vi "ReadMessage.vi"(8 "error in (no error)":errorcluster, 11 "StepMotor in":refnum<class "StepMotor.lvclass">) -> (0 "error out":errorcluster, 3 "StepMotor out":refnum<class "StepMotor.lvclass">)   [LabVIEW 2010, in "StepMotor.lvclass"]
doc: "Чтение сообщения из привода СПШ"
uses:
  StepMotor.lvclass
  StepMotor.lvclass/StepMotor.ctl
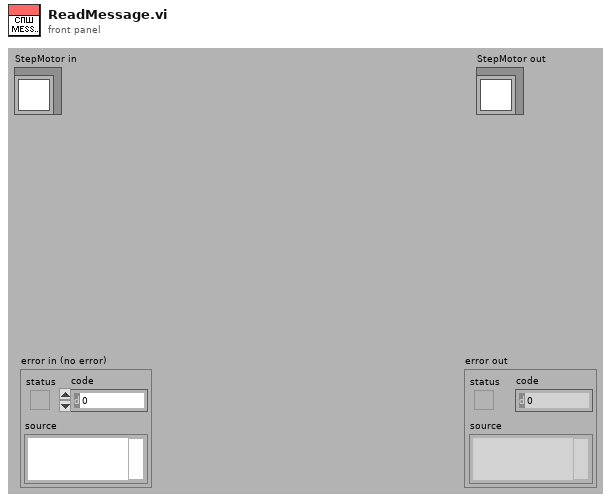
[diagram p1: front panel]
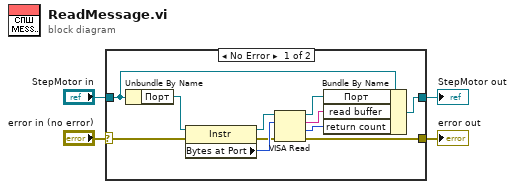
[diagram p0: block diagram]
diagram:
  n1 = case shown="No Error" "error in (no error)" {
    selector: "error in (no error)" -> [w6 w17]
    tunnel: [w8 w17] -> w3
    tunnel: [w14 w16] -> w1
    tunnel: "StepMotor in" -> [w15 w16]
    frame No Error {
      n2 = Unbundle By Name(w15) -> ("Порт"=w5:refnum<visa-resource-name>)
      n3 = property class="Instr"(reference=w5, error in=w6) -> (reference out=w11:refnum<visa-resource-name>, error out=w7:errorcluster, "Bytes at Port"=w10:u32)
      n4 = VISA Read(VISA resource name=w11, byte count=w10, error in (no error)=w7) -> (VISA resource name out=w13:refnum<visa-resource-name>, read buffer=w12:string, return count=w9:u32, error out=w8:errorcluster)
      n5 = Bundle By Name(cluster=w15, "Порт"=w13, "read buffer"=w12, "return count"=w9) -> (w14:refnum<class "StepMotor.lvclass">)
    }
    frame Error {
    }
  }
  "error out" <- w3
  "StepMotor out" <- w1
